vi "MagnaDC_Set Voltage.vi"(8 "error in (no error)":errorcluster, 11 "VISA resource name":refnum<visa-resource-name>="TCPIP0::131.227.181.163::50505::SOCKET") -> (0 "error out":errorcluster)   [LabVIEW 2022 SP3]
doc: "Simple example how to control power supplu output using voltage and current levels."
uses:
  Magna sub vis/MagnaDC.lvlib
panel:
  in  "Voltage Level (0.0 V)":dbl format="%.2g"
  # "(c) 2004 - 2018 Magna-Power Electronics Inc.  ALL RIGHTS RESERVED."
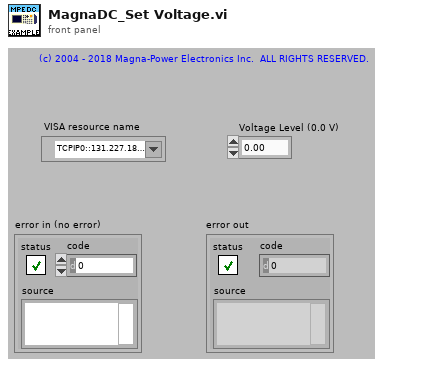
[diagram p1: front panel]
types:
  T1 = enum8{"Enabled", "Disabled", "Disabled and Grayed Out"}
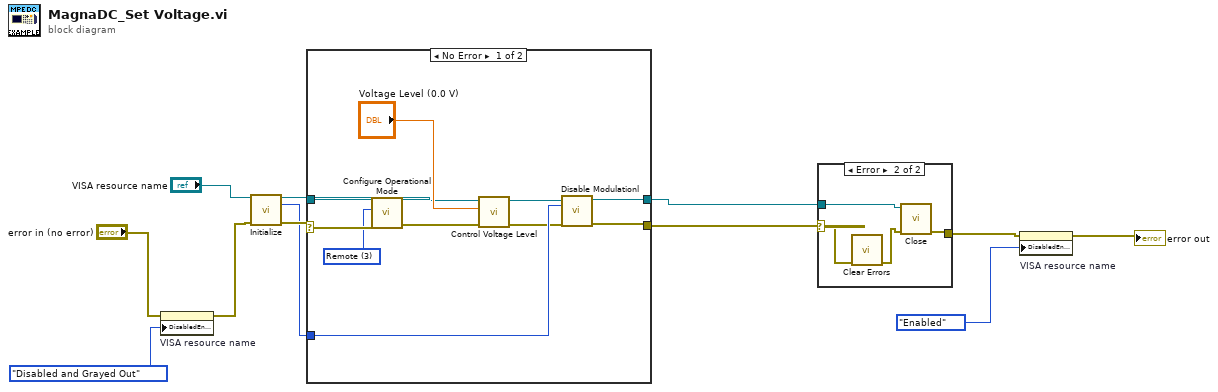
[diagram p0: block diagram]
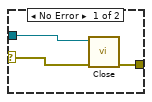
[diagram p2: hidden frame]
diagram:
  n1 = property on="VISA resource name" class="VISAName"(error in="error in (no error)", "DisabledEnum"=T1."Disabled and Grayed Out" ("Disabled")) -> (error out=w3:errorcluster)  [unwired: 1 in, 1 out]
  n2 = call "Initialize.vi"("VISA resource name"="VISA resource name", "error in (no error)"=w3) -> ("VISA resource name out"=w10:refnum<visa-resource-name>, "Modulation Available"=w1:u32, "error out"=w11:errorcluster)  [unwired: 10 in, 1 out]
  n3 = case shown="No Error" w11 {
    selector: w11 -> [w22 w25]
    tunnel: w10 -> [w23 w24]
    tunnel: [w18 w25] -> w8
    tunnel: [w19 w24] -> w7
    tunnel: w1 -> [w21 _]
    frame No Error {
      w20 = u32 3 items=["Rotary", "Keypad", "Ext Pgm", "Remote"] ("Operational Mode")
      n4 = call "Configure Operational Mode.vi"("error in (no error)"=w22, "Operational Mode"=w20, "VISA resource name"=w23) -> ("error out"=w15:errorcluster, "VISA resource name out"=w16:refnum<visa-resource-name>)  [unwired: 7 in]
      n5 = call "Control Voltage Level.vi"("error in (no error)"=w15, "Voltage Level (0.0 V)"="Voltage Level (0.0 V)", "VISA resource name"=w16) -> ("error out"=w14:errorcluster, "VISA resource name out"=w13:refnum<visa-resource-name>)  [unwired: 7 in]
      n6 = call "Disable Modulationl.vi"("VISA resource name"=w13, "Modulation"=w21, "error in (no error)"=w14) -> ("VISA resource name out"=w19:refnum<visa-resource-name>, "error out"=w18:errorcluster)  [unwired: 11 in]
    }
    frame Error {
    }
  }
  n7 = case shown="Error" w8 {
    selector: w8 -> [w28 w32]
    tunnel: [w26 w30] -> w6
    tunnel: w7 -> [w27 w29]
    frame No Error {
      n8 = call "Close.vi"("error in (no error)"=w28, "VISA resource name"=w27) -> ("error out"=w26:errorcluster)  [unwired: 9 in]
    }
    frame Error {
      n9 = call <vilib>:"Clear Errors.vi"("error in (no error)"=w32) -> ("error out"=w31:errorcluster)  [unwired: 5 in, 1 out]
      n10 = call "Close.vi"("error in (no error)"=w31, "VISA resource name"=w29) -> ("error out"=w30:errorcluster)  [unwired: 9 in]
    }
  }
  n11 = property on="VISA resource name" class="VISAName"(error in=w6, "DisabledEnum"=T1."Enabled" ("Disabled")) -> (error out=→"error out":errorcluster)  [unwired: 1 in, 1 out]
